vi "Image_Save_Dequeue_2.0.vi"(0 "Data":T1={"Camera 1"={"Camera1"="", "Cam 1"=FALSE, "CAM1 Model"=enum."a2A5328-15ucBAS", "Cam1 ID"=0}, "Camera 2"={"Camera2"="", "Cam 2"=FALSE, "CAM2 Model"=enum."a2A5328-15ucBAS", "Cam2 ID"=0}, "Image"={"Camera1_Img"=refnum, "Camera2_Img"=refnum, "Img1_Orig_Disp"=refnum, "Img2_Orig_Disp"=refnum, "Img1_Orig_RGB"=refnum, "Img2_Orig_RGB"=refnum, "Blue_Plane_Extract"=refnum, "Subtracted_Plane"=refnum, "Img1_Binary"=refnum, "Img2_Binary"=refnum, "Crop_Mask"=refnum, "Img1_Save"=refnum, "Img2_Save"=refnum, "Img1_Cali_Full"=refnum, "Img2_Cali_Full"=refnum, "Img1_Cali_Detect"=refnum, "Img2_Cali_Detect"=refnum}, "Ques"={"Cam 1 queue"=refnum, "Cam 2 queue"=refnum, "Cam 1 - save queue"=refnum, "Cam 2 - save queue"=refnum, "Image Process Queue Size"=500, "Image Save Queue Size"=500, "Overload threshold"=500, "Max large object threshold"=0}, "Arduino SRS"={"Pinch-valve"="", "Actuator"=FALSE, "Open(T)/Close(F)"=FALSE, "Arduino Uno"=""}, "Pump"={"Port"="", "Connection"=FALSE, "Flush Size"=0, "Command"="", "Pump Size"=enum."Large", "Pump"="", "Ready"=FALSE}, "Camera settings"={"Detection settings"={"Sample size threshold"=500, "Detection Region %"=30.0, "Timeout Sample"=200}, "Lens/camera settings"={"Aperture"=enum."Item 0", "Legacy Cam Attributes"=FALSE, "Max Framerate"=100, "Exposure Time"=1000.0, "Framerate"=15}, "Crop settings"={"Cam1"={"Rectangle 1"={"Left"=0, "Top"=0, "Right"=0, "Bottom"=0, "Rotation"=0.0}, "Camera Orientation 1"="", "Pixel to mm 1"=0.0}, "Cam2"={"Rectangle 2"={"Left"=0, "Top"=0, "Right"=0, "Bottom"=0, "Rotation"=0.0}, "Camera Orientation 2"="", "Pixel to mm 2"=0.0}}}, "Arduino ISS"={"Mega F3"="", "Phase3"=FALSE, "Barcode"="", "Sorting sys."=FALSE, "Initial size"=0.0, "Size Interval"=0.0, "Mun. of containers"=0.0, "Container nr."=0.0, "Arduino Mega"=""}, "Img_Capt"=FALSE, "Empty_Refill"=FALSE, "I don't think is in use"={"Light intensity"=100}, "Extended setup"={"Location"="Station", "Latitude"="Station", "Longitude"="Station", "Determiner"="Station", "Sex"="Station", "Station"="", "Collection date"=""}, "Main interface"={"Sample Name"="Test Sample", "Operator"="JFR", "Species Name"="", "Other Notes"=""}, "Tap1"=0, "SystemVersion"=0, "System Serial"="", "Exit"=FALSE, "Kuvette Full"=FALSE, "Core JKI"={"Current VI Reference"=refnum, "Close Panel on Exit?"=FALSE}, "Calibration"={"Calibration 1"=path "C:/Users/au540322/Desktop/IHS_Project/images/Debris/Debris_0/Debris_0_2019_06_01-23-32-49-686.PNG", "Calibration 2"=path "C:/Users/au540322/Desktop/IHS_Project/images/Debris/Debris_0/Debris_0_2019_06_01-23-32-49-686.PNG", "Detect 1"=path "C:/Users/au540322/Desktop/IHS_Project/images/Debris/Debris_0/Debris_0_2019_06_01-23-32-49-686.PNG", "Detect 2"=path "C:/Users/au540322/Desktop/IHS_Project/images/Debris/Debris_0/Debris_0_2019_06_01-23-32-49-686.PNG"}, "Auto Flush"=FALSE, "Status History"="", "Timestamp Start"=""} {"SystemVersion" items=["Standard", "XL"]; "Tap1" items=["Session Data", "Extended Setup", "Buffer", "Camera", "Dispenser", "Stats", "Connections"]; "I don't think is in use"."Light intensity" scale=0.0..100.0; "Camera settings"."Crop settings"."Cam2"."Rectangle 2"."Rotation" format="%.2f"; "Camera settings"."Crop settings"."Cam2"."Rectangle 2"."Left" scale=0.0..1024.0; "Camera settings"."Crop settings"."Cam2"."Rectangle 2"."Right" scale=0.0..1024.0; "Camera settings"."Crop settings"."Cam1"."Rectangle 1"."Rotation" format="%.2f"; "Camera settings"."Crop settings"."Cam1"."Rectangle 1"."Left" scale=0.0..1024.0; "Camera settings"."Crop settings"."Cam1"."Rectangle 1"."Right" scale=0.0..1024.0; "Camera settings"."Lens/camera settings"."Framerate" min=1; "Camera settings"."Lens/camera settings"."Max Framerate" min=1; "Camera settings"."Detection settings"."Sample size threshold" min=1; "Pump"."Flush Size" min=0 max=6000 step=100; "Ques"."Overload threshold" min=1; "Ques"."Image Save Queue Size" min=1; "Ques"."Image Process Queue Size" min=1}, 2 "Camera":T5, 3 "Old":i32, 4 "cam1_prev":u32, 5 "Other":i32, 6 "Queue active":bool, 7 "cam2_prev":u32) -> (16 "timed out?":bool, 17 "Sample Data":dbl[](array[numeric]), 20 "# elements in queue":i32, 22 "State out":i32, 23 "Image Save 1":T3, 24 "cam1_count":u32, 25 "Image Save 2":T3, 26 "Last image":bool, 27 "cam2_count":u32)   [LabVIEW 2024]
uses:
  Camera_ID.ctl
  <vilib>/vision/Image Controls.llb/IMAQ Image.ctl
  controls/Data_JKI.ctl
  <vilib>/userDefined/High Color/IMAQdx.ctl
panel:
  out "error out 3":errorcluster
  out "error out 2":errorcluster
  out "error out":errorcluster
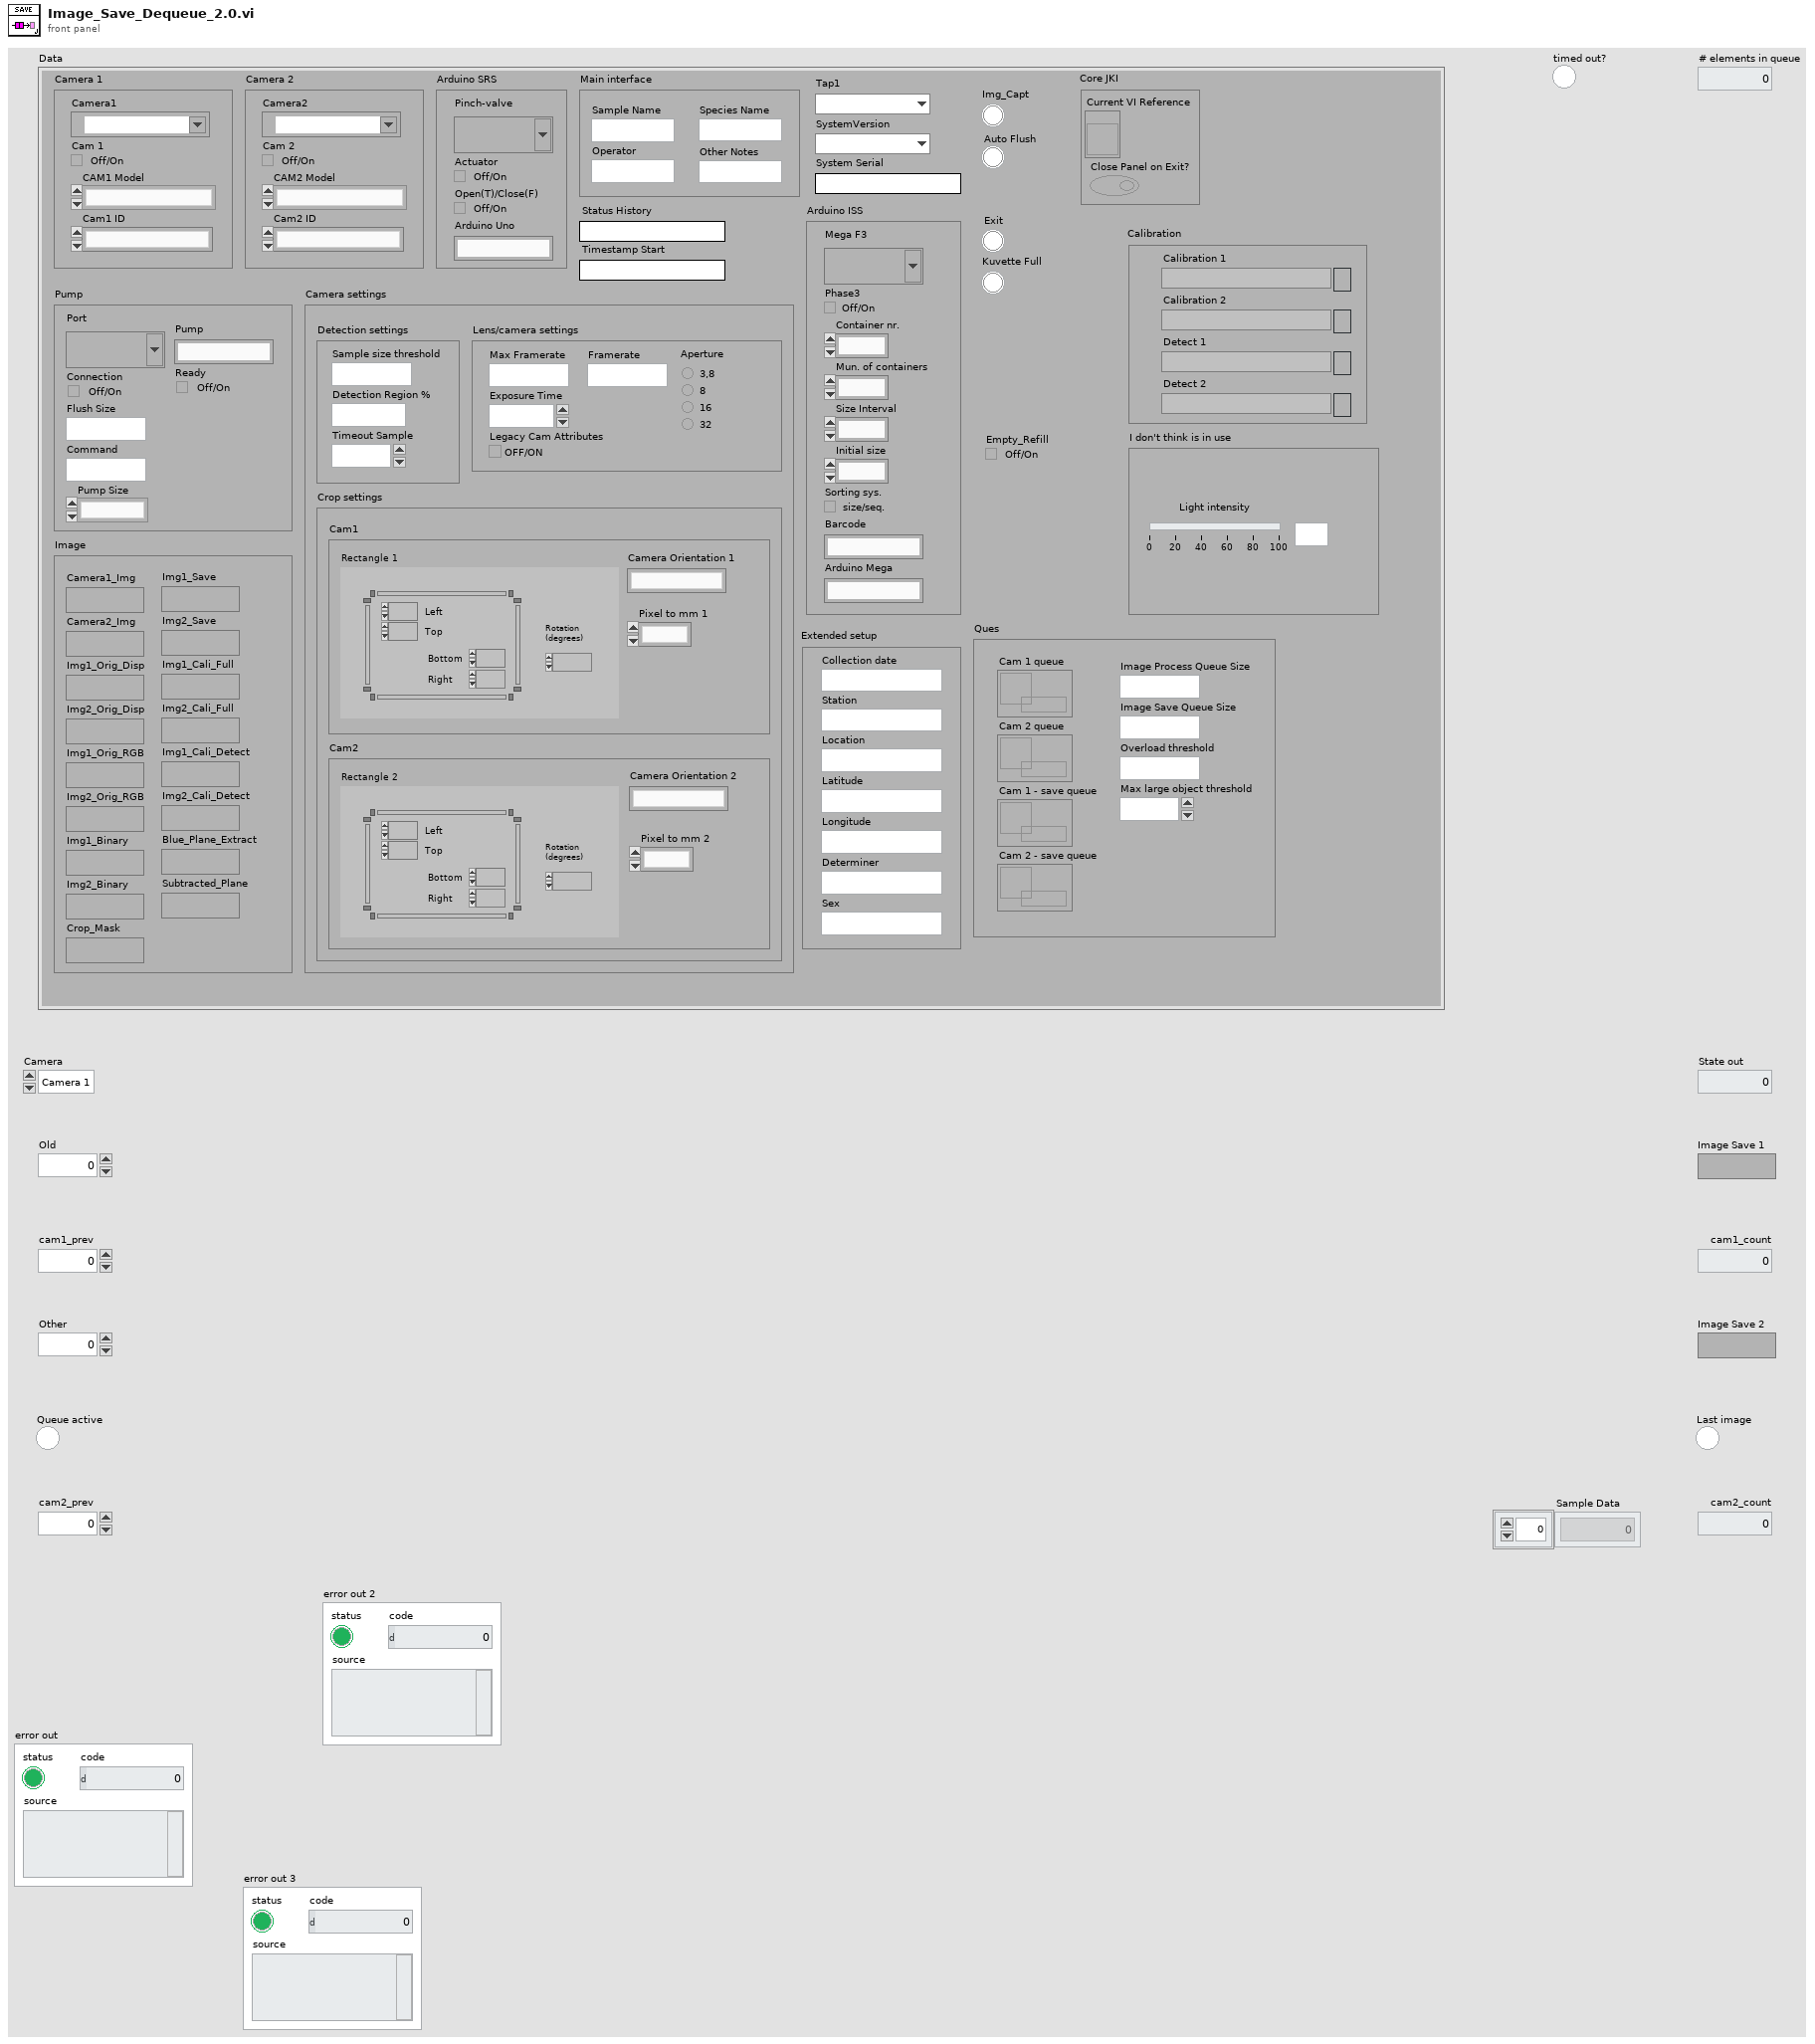
[diagram p1: front panel]
types:
  T1 = typedef "Data_JKI.ctl" = cluster{"Camera 1":cluster{"Camera1":T2, "Cam 1":bool, "CAM1 Model":enum16{"a2A5328-15ucBAS", "acA1920-155uc"}, "Cam1 ID":i32}, "Camera 2":cluster{"Camera2":T2, "Cam 2":bool, "CAM2 Model":enum16{"a2A5328-15ucBAS", "acA1920-155uc"}, "Cam2 ID":i32}, "Image":cluster{"Camera1_Img":T3, "Camera2_Img":T3, "Img1_Orig_Disp":T3, "Img2_Orig_Disp":T3, "Img1_Orig_RGB":T3, "Img2_Orig_RGB":T3, "Blue_Plane_Extract":T3, "Subtracted_Plane":T3, "Img1_Binary":T3, "Img2_Binary":T3, "Crop_Mask":T3, "Img1_Save":T3, "Img2_Save":T3, "Img1_Cali_Full":T3, "Img2_Cali_Full":T3, "Img1_Cali_Detect":T3, "Img2_Cali_Detect":T3}, "Ques":cluster{"Cam 1 queue":refnum<queue>, "Cam 2 queue":refnum<queue>, "Cam 1 - save queue":refnum<queue>, "Cam 2 - save queue":refnum<queue>, "Image Process Queue Size":i32, "Image Save Queue Size":i32, "Overload threshold":i32, "Max large object threshold":i32}, "Arduino SRS":cluster{"Pinch-valve":refnum<visa-resource-name>, "Actuator":bool, "Open(T)/Close(F)":bool, "Arduino Uno":string}, "Pump":cluster{"Port":refnum<visa-resource-name>, "Connection":bool, "Flush Size":i32, "Command":string, "Pump Size":enum16{"None", "Small", "Large"}, "Pump":string, "Ready":bool}, "Camera settings":cluster{"Detection settings":cluster{"Sample size threshold":i32, "Detection Region %":dbl, "Timeout Sample":i32}, "Lens/camera settings":cluster{"Aperture":enum32{"Item 0", "Item 1", "Item 2", "Item 3"}, "Legacy Cam Attributes":bool, "Max Framerate":i32, "Exposure Time":dbl, "Framerate":i32}, "Crop settings":cluster{"Cam1":cluster{"Rectangle 1":T4, "Camera Orientation 1":string, "Pixel to mm 1":dbl}, "Cam2":cluster{"Rectangle 2":T4, "Camera Orientation 2":string, "Pixel to mm 2":dbl}}}, "Arduino ISS":cluster{"Mega F3":refnum<visa-resource-name>, "Phase3":bool, "Barcode":string, "Sorting sys.":bool, "Initial size":dbl, "Size Interval":dbl, "Mun. of containers":dbl, "Container nr.":dbl, "Arduino Mega":string}, "Img_Capt":bool, "Empty_Refill":bool, "I don't think is in use":cluster{"Light intensity":i32}, "Extended setup":cluster{"Location":string, "Latitude":string, "Longitude":string, "Determiner":string, "Sex":string, "Station":string, "Collection date":string}, "Main interface":cluster{"Sample Name":string, "Operator":string, "Species Name":string, "Other Notes":string}, "Tap1":u16, "SystemVersion":u16, "System Serial":string, "Exit":bool, "Kuvette Full":bool, "Core JKI":cluster{"Current VI Reference":refnum<vi>, "Close Panel on Exit?":bool}, "Calibration":cluster{"Calibration 1":path, "Calibration 2":path, "Detect 1":path, "Detect 2":path}, "Auto Flush":bool, "Status History":string, "Timestamp Start":string}
  T2 = typedef "IMAQdx.ctl" = refnum<k21>
  T3 = typedef "IMAQ Image.ctl" = refnum<image>
  T4 = typedef "IMAQ Rectangle" = cluster{"Left":i32, "Top":i32, "Right":i32, "Bottom":i32, "Rotation":dbl}
  T5 = typedef "Camera_ID.ctl" = enum16{"Camera 1", "Camera 2"}
  T6 = cluster{"Timestamp":string, "Image Pixels (U32)":u32[][], "Prev. sample":i32, "Sample Data":dbl[], "output cluster":cluster{"Global Rectangle":i32[], "Contours":cluster{"ID":enum32{"External", "Internal"}, "Type":u32, "Coordinates":i32[]}[]}}
  T7 = cluster{"Global Rectangle":i32[], "Contours":cluster{"ID":enum32{"External", "Internal"}, "Type":u32, "Coordinates":i32[]}[]}
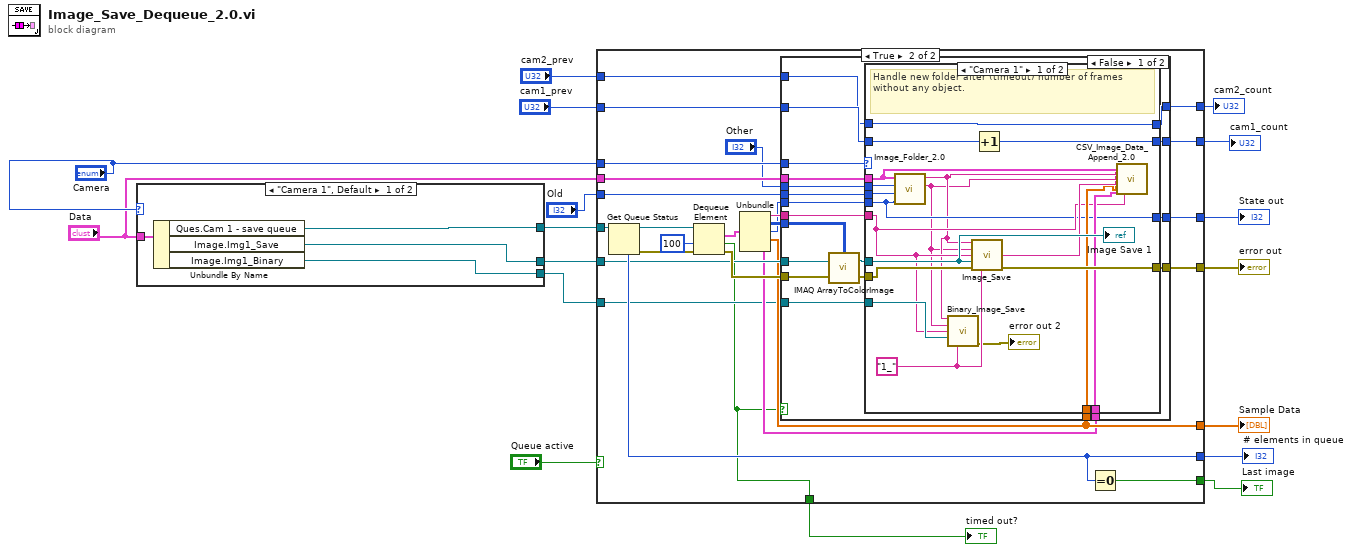
[diagram p0: block diagram]
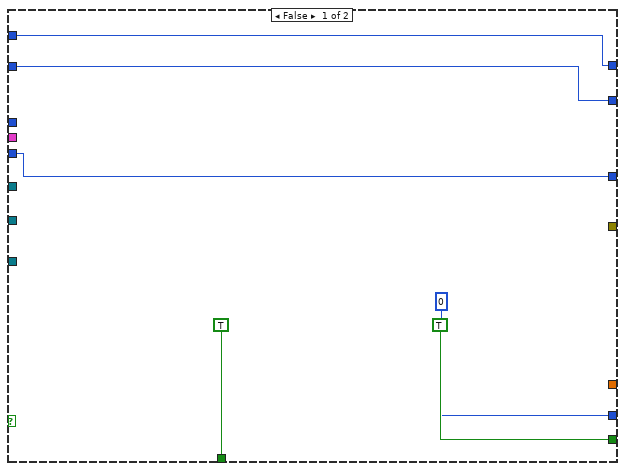
[diagram p2: hidden frame]
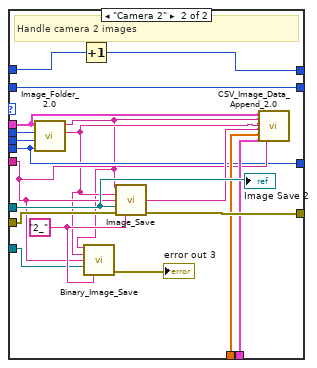
[diagram p3: hidden frame]
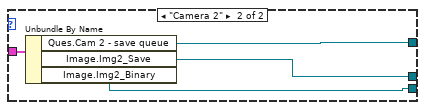
[diagram p5: hidden frame]
diagram:
  n1 = case shown="\"Camera 1\", Default" "Camera" {
    tunnel: [w20 w25] -> w16
    tunnel: "Data" -> [w21 w24]
    tunnel: [w19 w23] -> w7
    tunnel: [w18 w22] -> w2
    frame "Camera 1", Default {
      n2 = Unbundle By Name(w21) -> ("Ques.Cam 1 - save queue"=w20:refnum<queue>, "Image.Img1_Save"=w19:T3, "Image.Img1_Binary"=w18:T3)
    }
    frame "Camera 2" {
      n3 = Unbundle By Name(w24) -> ("Ques.Cam 2 - save queue"=w25:refnum<queue>, "Image.Img2_Save"=w23:T3, "Image.Img2_Binary"=w22:T3)
    }
  }
  n4 = case shown="True" "Queue active" {
    tunnel: "Camera" -> [_ w57]
    tunnel: w16 -> [_ w53]
    tunnel: "Data" -> [_ w52]
    tunnel: [0 ("# elements in queue") w51] -> w14
    tunnel: [TRUE w50] -> w13
    tunnel: [_ w49] -> w12
    tunnel: [w29 w44] -> w11
    tunnel: "Old" -> [w29 w43]
    tunnel: [_ w39] -> w9
    tunnel: [TRUE ("timed out?") w32] -> w8
    tunnel: w7 -> [_ w40]
    tunnel: [w27 w37] -> w6
    tunnel: "cam1_prev" -> [w27 w36]
    tunnel: "cam2_prev" -> [w26 w35]
    tunnel: [w26 w34] -> w3
    tunnel: w2 -> [_ w33]
    frame False {
    }
    frame True {
      n5 = Get Queue Status(queue=w53) -> (queue out=w54:refnum<queue>, error out=w47:errorcluster, # elements in queue=w51:i32)  [unwired: 2 in, 5 out]
      n6 = Dequeue Element(queue=w54, timeout in ms (-1)=100, error in (no error)=w47) -> (element=w56:T6, timed out?=w32:bool, error out=w41:errorcluster)  [unwired: 1 out]
      n7 = Unbundle(w56) -> ("Timestamp"=w48:string, "Image Pixels (U32)"=w55:u32[][], "Prev. sample"=w46:i32, "Sample Data"=w39:dbl[], "output cluster"=w38:T7)
      n8 = case shown="False" w32 {
        tunnel: w57 -> [w77 _]
        tunnel: w55 -> [w65 _]
        tunnel: w52 -> [w76 _]
        tunnel: [w75 w118] -> w49
        tunnel: w48 -> [w74 _]
        tunnel: w46 -> [w73 _]
        tunnel: "Other" -> [w72 _]
        tunnel: [w71 w119] -> w44
        tunnel: w43 -> [w70 w119]
        tunnel: w41 -> [w66 w118]
        tunnel: w40 -> [w69 _]
        tunnel: w39 -> [w64 _]
        tunnel: w38 -> [w63 _]
        tunnel: [w62 w117] -> w37
        tunnel: w36 -> [w61 w117]
        tunnel: w35 -> [w60 w116]
        tunnel: [w59 w116] -> w34
        tunnel: w33 -> [w58 _]
        frame False {
          n9 = call "IMAQ ArrayToColorImage"("Image Pixels (U32)"=w65, "Image"=w69, "error in (no error)"=w66) -> ("Image Out"=w68:T3, "error out"=w67:errorcluster)  [unwired: 2 in]
          n10 = case shown="\"Camera 1\"" w77 {
            tunnel: [w96 w115] -> w75
            tunnel: w68 -> [w94 w113]
            tunnel: w76 -> [w83 w102]
            tunnel: w74 -> [w84 w103]
            tunnel: w67 -> [w95 w114]
            tunnel: w73 -> [w80 w99]
            tunnel: w70 -> [w81 w100]
            tunnel: w72 -> [w82 w101]
            tunnel: [w80 w99] -> w71
            tunnel: w64 -> [w86 w105]
            tunnel: w63 -> [w85 w104]
            tunnel: [w93 w110] -> w62
            tunnel: w61 -> [w92 w110]
            tunnel: w60 -> [w91 w112]
            tunnel: [w91 w111] -> w59
            tunnel: w58 -> [w90 w108]
            frame "Camera 1" {
              w89 = "1_" ("Camera image prefix")
              # "Handle new folder after (timeout) number of frames without any object."
              n11 = call "Image_Folder_2.0.vi"("New"=w80, "Old"=w81, "Other"=w82, "Data"=w83) -> ("Subfolder Name"=w78:string, "Subfolder Path"=w79:string)  [unwired: 6 in]
              n12 = call "Binary_Image_Save.vi"("Subfolder path"=w79, "Subfolder Name"=w78, "Timestamp"=w84, "Image in"=w90, "Camera"=w89) -> ("error out"=→"error out 2":errorcluster)  [unwired: 7 in, 3 out]
              n13 = call "Image_Save.vi"("Subfolder path"=w79, "Subfolder Name"=w78, "Timestamp"=w84, "Image in"=w94, "error in"=w95, "Camera"=w89) -> ("Image Name"=w87:string, "error out"=w96:errorcluster)  [unwired: 6 in, 2 out]
              n14 = Increment(x=w92) -> (x+1=w93:u32)
              n15 = call "CSV_Image_Data_Append_2.0.vi"("Data"=w83, "Image path"=w79, "Sample Name"=w78, "Image Name"=w87, "Sample Data"=w86, "ROI Descriptor"=w85, "Timestamp"=w84) -> ()  [unwired: 13 in]
              "Image Save 1" <- w94
            }
            frame "Camera 2" {
              w109 = "2_" ("Camera image prefix")
              # "Handle camera 2 images"
              n16 = call "Image_Folder_2.0.vi"("New"=w99, "Old"=w100, "Other"=w101, "Data"=w102) -> ("Subfolder Name"=w98:string, "Subfolder Path"=w97:string)  [unwired: 6 in]
              n17 = Increment(x=w112) -> (x+1=w111:u32)
              n18 = call "Binary_Image_Save.vi"("Subfolder path"=w97, "Subfolder Name"=w98, "Timestamp"=w103, "Image in"=w108, "Camera"=w109) -> ("error out"=→"error out 3":errorcluster)  [unwired: 7 in, 3 out]
              n19 = call "Image_Save.vi"("Subfolder path"=w97, "Subfolder Name"=w98, "Timestamp"=w103, "Image in"=w113, "error in"=w114, "Camera"=w109) -> ("Image Name"=w106:string, "error out"=w115:errorcluster)  [unwired: 6 in, 2 out]
              n20 = call "CSV_Image_Data_Append_2.0.vi"("Data"=w102, "Image path"=w97, "Sample Name"=w98, "Image Name"=w106, "Sample Data"=w105, "ROI Descriptor"=w104, "Timestamp"=w103) -> ()  [unwired: 13 in]
              "Image Save 2" <- w113
            }
          }
        }
        frame True {
        }
      }
      n21 = Equal To 0?(x=w51) -> (x = 0?=w50:bool)
    }
  }
  "# elements in queue" <- w14
  "Last image" <- w13
  "error out" <- w12
  "State out" <- w11
  "Sample Data" <- w9
  "timed out?" <- w8
  "cam1_count" <- w6
  "cam2_count" <- w3
